vi "Get_Inst_Index.vi"(10 "Inst name search":string, 11 "Analysis Info cluster":T1[](array[typedef])) -> (0 "Success":bool, 2 "Index of Instance":i32, 3 "Inst Name Array":string[](array[string]))   [LabVIEW 2011]
uses:
  Controls/Analysis_info_cluster.ctl
  Controls/Inst_type.ctl
  Controls/Instrument_Array.ctl
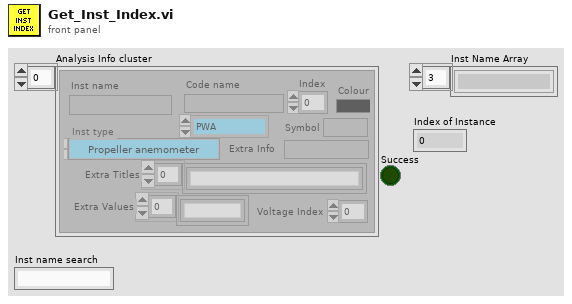
[diagram p1: front panel]
types:
  T1 = typedef "Analysis_info_cluster.ctl" = cluster{"Colour":u32, "Inst type":T2, "Inst name":string, "Symbol":string, "Code name":string, "Extra Info":string, "Inst Array":T3, "Index":i32, "Voltage Index":i32, "Extra Titles":string[], "Extra Values":string[]}
  T2 = typedef "Inst_type.ctl" = enum16{"Propeller anemometer", "Raw voltage", "Pressure Transducer", "Pitot-static tube", "Preston tube", "Hot wire", "Cross wire 1", "Cross wire 2", "Generic Linear", "Generic Polynomial", "Generic BackPoly", "Fast FID", "Thermocouple", "Cold wire", "Pulsed Wire", "LDA Vel", "LDA Tran time", "LDA Arr time"}
  T3 = typedef "Instrument_Array.ctl" = enum16{"PWA", "LDA", "Analogue"}
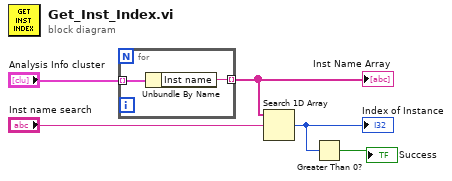
[diagram p0: block diagram]
diagram:
  n1 = for {
    tunnel: "Analysis Info cluster" -> [w7] mode=indexing
    tunnel: [w6] -> w5 mode=indexing
    n2 = Unbundle By Name(w7) -> ("Inst name"=w6:string)
  }
  "Inst Name Array" <- w5
  n3 = Search 1D Array(1D array=w5, element="Inst name search") -> (index of element=w2:i32)  [unwired: 1 in]
  "Index of Instance" <- w2
  n4 = Greater Than 0?(x=w2) -> (x > 0?=→"Success":bool)
